vi "archive.request.vi"(8 "error in":errorcluster) -> (0 "error out":errorcluster, 1 "Request":string)   [LabVIEW 2020, in "asset.lvclass"]
uses:
  asset.lvclass
  asset.lvclass/asset.ctl
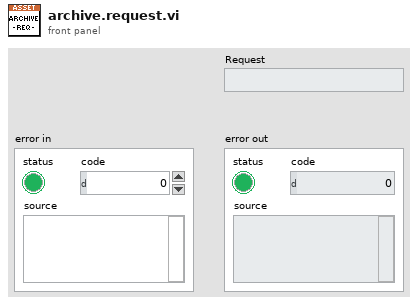
[diagram p1: front panel]
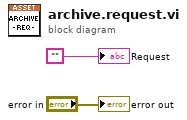
[diagram p0: block diagram]
diagram:
  "Request" <- ""
  "error out" <- "error in"
